vi "Stop BuildWorker.vi"(8 "error in (no error)":errorcluster, 11 "BuildWorker Basics in":refnum<class "BuildWorker Basics.lvclass">) -> (0 "error out":errorcluster, 3 "BuildWorker Basics out":refnum<class "BuildWorker Basics.lvclass">)   [LabVIEW 2017, in "BuildWorker Interface.lvlib" / "BuildWorker Basics.lvclass"]
uses:
  BuildWorker Basics.lvclass
  <vilib>/ActorFramework/Stop Msg/Stop Msg.lvclass
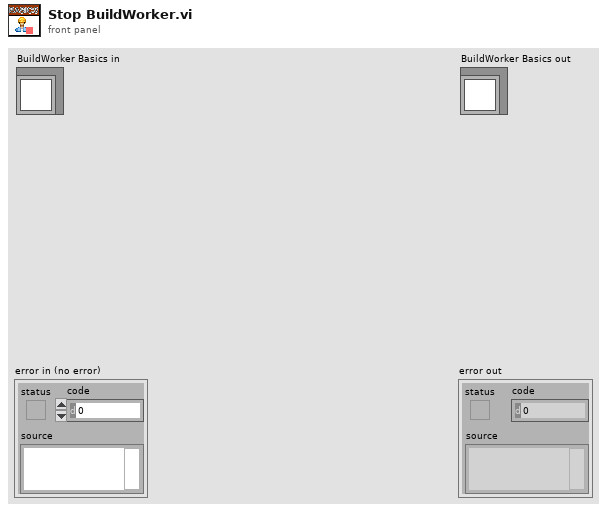
[diagram p1: front panel]
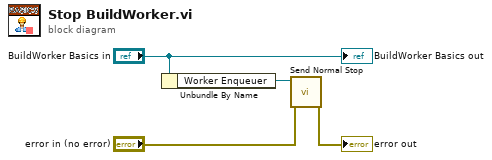
[diagram p0: block diagram]
diagram:
  n1 = Unbundle By Name("BuildWorker Basics in") -> ("Worker Enqueuer"=w3:refnum<class "Message Enqueuer.lvclass">)
  n2 = call <vilib>:"Send Normal Stop.vi"("error in (no error)"="error in (no error)", "Message Enqueuer"=w3) -> ("error out"=→"error out":errorcluster)  [unwired: 9 in]
  "BuildWorker Basics out" <- "BuildWorker Basics in"
